vi "数组的创建.vi"() -> ()   [LabVIEW 2018]
panel:
  out "数组 3":i32[][](array[numeric])
  out "数组 2":i32[](array[numeric])
  out "添加的数组":dbl[](array[numeric])
  in  "元素 5":dbl
  in  "元素 4":dbl
  in  "元素 3":dbl
  in  "元素 2":dbl
  in  "元素":dbl
  out "初始化的数组":dbl[](array[numeric])
  in  "数组":bool[][][](array[boolean])
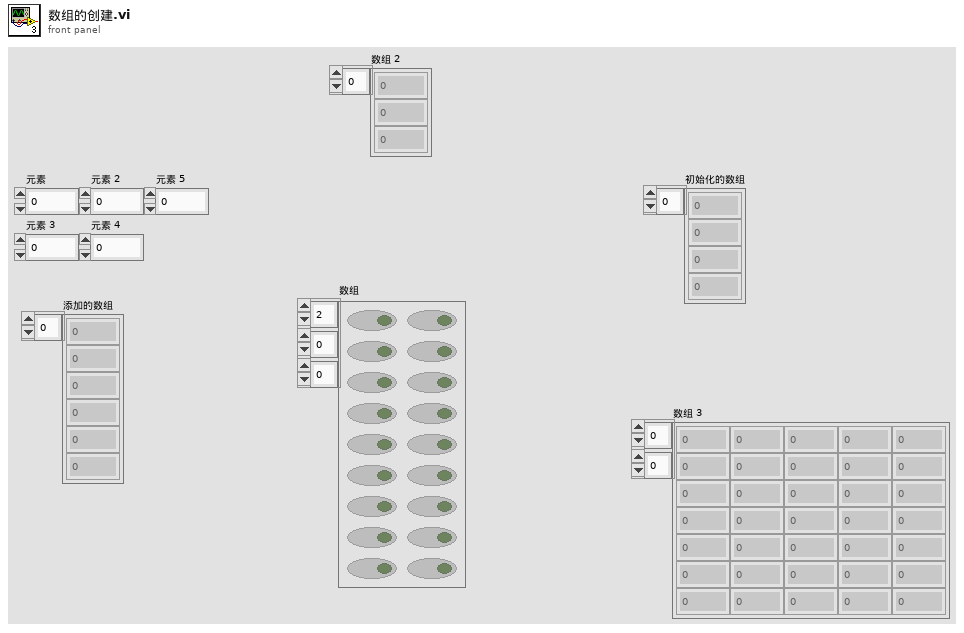
[diagram p1: front panel]
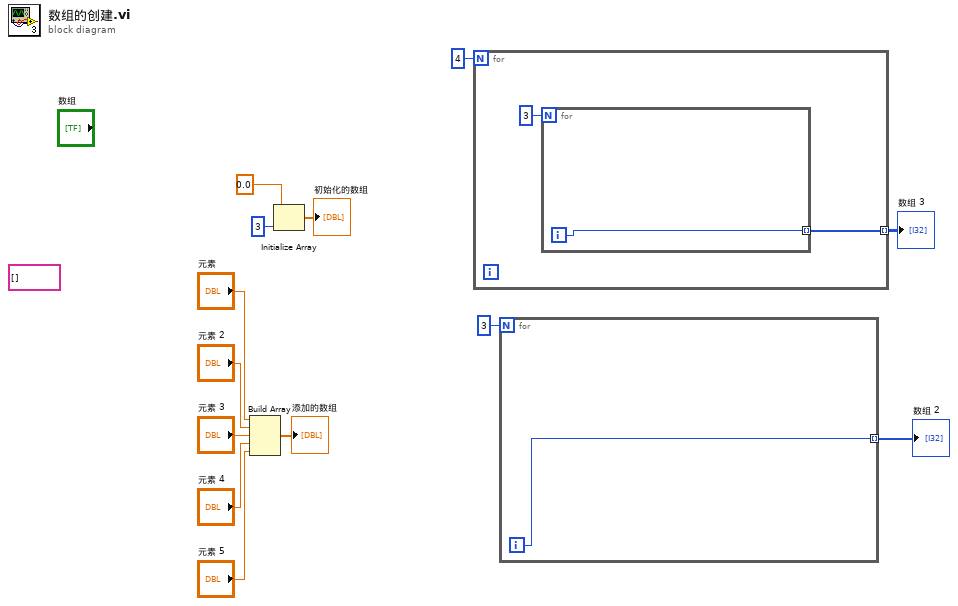
[diagram p0: block diagram]
diagram:
  (unwired) string[] []
  n1 = Build Array("元素", "元素 2", "元素 3", "元素 4", "元素 5") -> (→"添加的数组":dbl[])
  n2 = Initialize Array(0.0 ("元素"), 3 ("维数大小")) -> (→"初始化的数组":dbl[])
  n3 = for {
    N: 4 -> [_]
    tunnel: [w14] -> w1 mode=indexing
    n4 = for {
      N: 3 -> [_]
      tunnel: [w16] -> w14 mode=indexing
      i -> [w16]
    }
  }
  "数组 3" <- w1
  n5 = for {
    N: 3 -> [_]
    tunnel: [w17] -> w3 mode=indexing
    i -> [w17]
  }
  "数组 2" <- w3
